vi "FGPA_Main_test.vi"() -> ()   [LabVIEW 2017]
uses:
  <vilib>/rvi/Emulation/niFpgaGetClockAttributes.vi
  <vilib>/rvi/Emulation/niFpgaSctlEmulationGetInTimedLoop.vi
  <vilib>/rvi/Emulation/niFpgaEmulationReportErrorSimple.vi
  <vilib>/rvi/Emulation/niFpgaCriticalErrorInLSC.vi
panel:
  out "Boolean Indicator":bool
  out "FXP Indicator":fxp<+/-,20,5>
  out "I32 Indicator":i32
  out "SGL Indicator":sgl
  in  "Boolean Control":bool
  in  "FXP Control":fxp<+/-,20,5>
  in  "I32 Control":i32
  in  "SGL Control":sgl
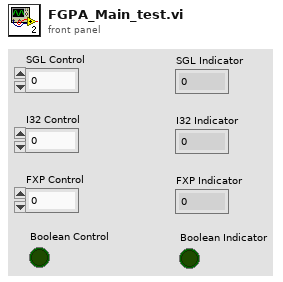
[diagram p1: front panel]
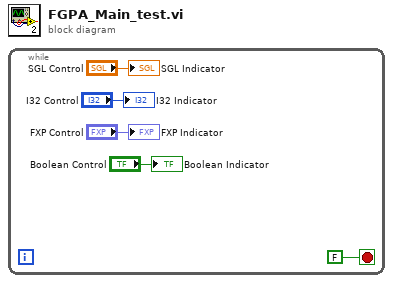
[diagram p0: block diagram]
diagram:
  n1 = while {
    stop <- FALSE stop-if-true
    "SGL Indicator" <- "SGL Control"
    "I32 Indicator" <- "I32 Control"
    "FXP Indicator" <- "FXP Control"
    "Boolean Indicator" <- "Boolean Control"
  }
